vi "File.String Array to CSV_V2.vi"(8 "error in":errorcluster, 9 "2D Array":string[][](array[string]), 10 "Top Row (Header)":string[](array[string]), 11 "File":path=path "C:/Users/eddiek/Documents/01_MTE/Circle Test/Results/ATS_TL/Circle Test Summary Data, 10-06-2017/AB736001B5_CT02_CS01.csv") -> (0 "error out":errorcluster, 3 "Dup File":path)   [LabVIEW 2018]
uses:
  <vilib>/KATE/Files/File Utils.lvlib
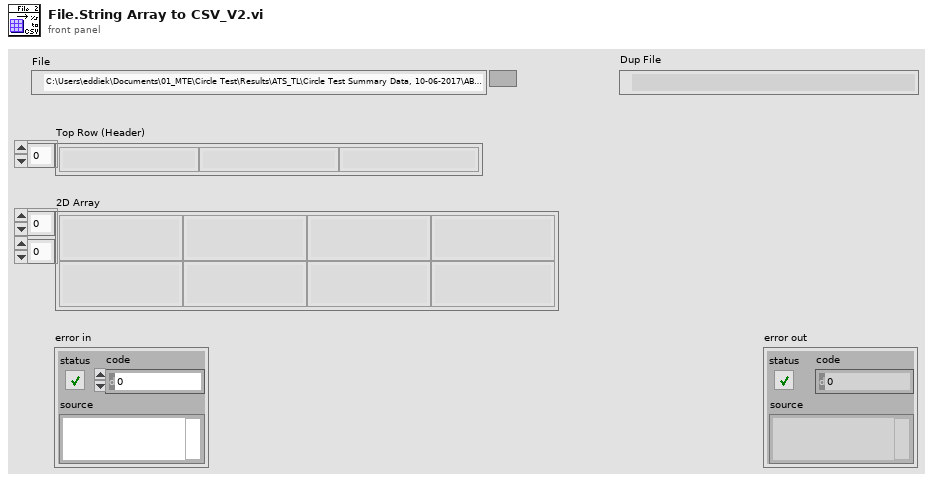
[diagram p1: front panel]
types:
  T1 = enum16{"open", "replace", "create", "open or create", "replace or create", "replace or create with confirmation"}
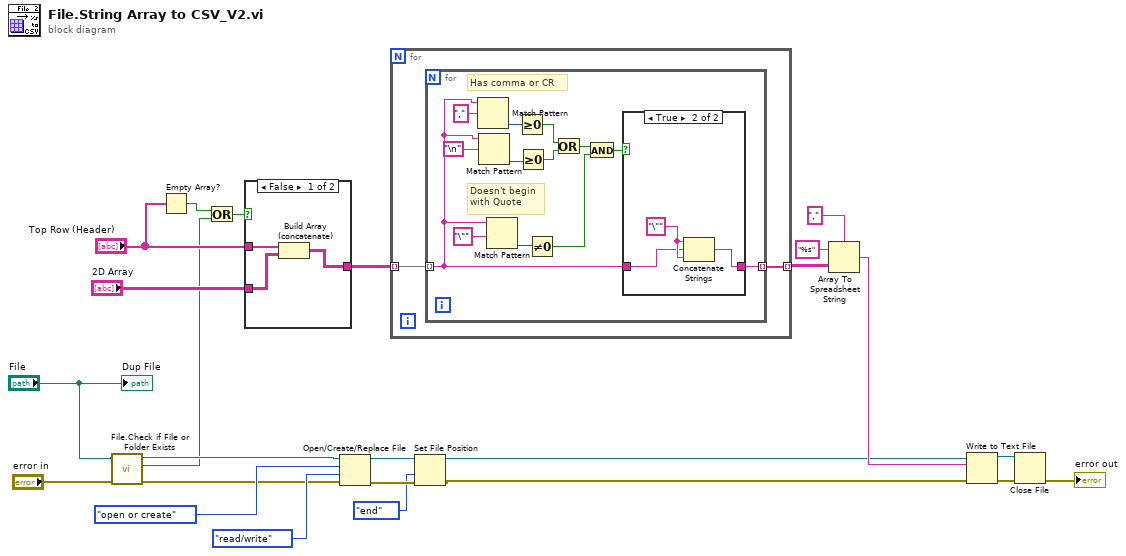
[diagram p0: block diagram]
diagram:
  n1 = call <vilib>:"File.Check if File or Folder Exists.vi"("error in"="error in", "Path"="File") -> ("error out"=w9:errorcluster, "Exists"=w6:bool, "Dup Path"=w11:path)  [unwired: 5 in, 2 out]
  n2 = Empty Array?(array="Top Row (Header)") -> (empty?=w7:bool)
  n3 = Or(x=w7, y=w6) -> (x .or. y?=w8:bool)
  n4 = case shown="False" w8 {
    tunnel: "Top Row (Header)" -> [w27 _]
    tunnel: "2D Array" -> [w26 w28]
    tunnel: [w25 w28] -> w22
    frame False {
      n5 = Build Array (concatenate)(w27, w26) -> (w25:string[][])
    }
    frame True {
    }
  }
  n6 = Open/Create/Replace File(file path (use dialog)=w11, error in=w9, operation (0:open)=T1."open or create", access (0:read/write)=enum16{"read/write", "read-only", "write-only"}."read/write") -> (refnum out=w5:refnum<file>, error out=w4:errorcluster)  [unwired: 2 in, 1 out]
  n7 = for {
    tunnel: w22 -> [w30] mode=indexing
    tunnel: [w29] -> w21 mode=indexing
    n8 = for {
      tunnel: w30 -> [w31] mode=indexing
      tunnel: [w37] -> w29 mode=indexing
      # "Has comma or CR"
      # "Doesn't begin\nwith Quote"
      n9 = Match Pattern(string=w31, regular expression=",") -> (offset past match=w41:i32)  [unwired: 1 in, 3 out]
      n10 = Match Pattern(string=w31, regular expression="\n") -> (offset past match=w40:i32)  [unwired: 1 in, 3 out]
      n11 = Match Pattern(string=w31, regular expression="\"") -> (offset past match=w36:i32)  [unwired: 1 in, 3 out]
      n12 = Greater Or Equal To 0?(x=w41) -> (x >= 0?=w39:bool)
      n13 = Greater Or Equal To 0?(x=w40) -> (x >= 0?=w38:bool)
      n14 = Not Equal To 0?(x=w36) -> (x != 0?=w32:bool)
      n15 = Or(x=w39, y=w38) -> (x .or. y?=w33:bool)
      n16 = And(x=w33, y=w32) -> (x .and. y?=w34:bool)
      n17 = case shown="True" w34 {
        tunnel: w31 -> [w44 w46]
        tunnel: [w44 w45] -> w37
        frame False {
        }
        frame True {
          w47 = "\""
          n18 = Concatenate Strings(w47, w46, w47) -> (w45:string)
        }
      }
    }
  }
  n19 = Set File Position(refnum=w5, from (0:start)=enum16{"start", "end", "current"}."end", error in=w4) -> (refnum out=w1:refnum<file>, error out=w2:errorcluster)  [unwired: 1 in]
  n20 = Array To Spreadsheet String(delimiter (Tab)=",", array=w21, 3:"%s" ("format string")) -> (spreadsheet string=w18:string)
  n21 = Write to Text File(file (use dialog)=w1, text=w18, error in=w2) -> (refnum out=w16:refnum<file>, error out=w17:errorcluster)  [unwired: 1 in, 1 out]
  n22 = Close File(refnum=w16, error in=w17) -> (error out=→"error out":errorcluster)  [unwired: 1 out]
  "Dup File" <- "File"
